vi "CollectorWrap.vi"(7 "Action":T1=enum."Collect") -> ()   [LabVIEW 2013]
uses:
  CollectorWrapAction.ctl
  DoubleSolenoidAction.ctl
  Autonomous/RollerStates.ctl
panel:
  out "error out":errorcluster
  in  "error in":errorcluster
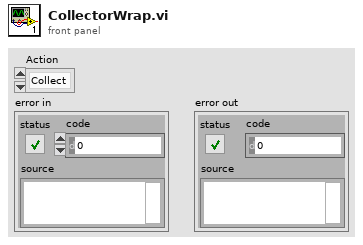
[diagram p1: front panel]
types:
  T1 = typedef "CollectorWrapAction.ctl" = enum16{"PreCollect", "Collect", "Stop"}
  T2 = typedef "DoubleSolenoidAction.ctl" = enum16{"Init", "Middle", "In", "Out"}
  T3 = typedef "RollerStates.ctl" = enum16{"Init", "Off", "Forward", "Reverse"}
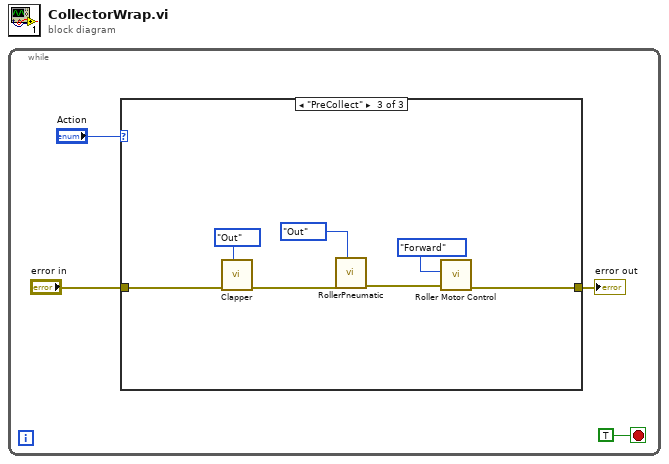
[diagram p0: block diagram]
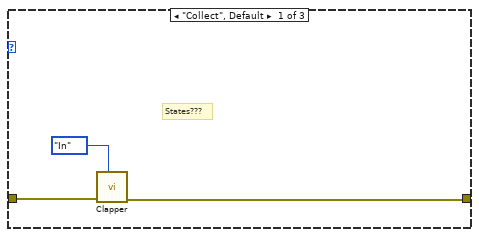
[diagram p2: hidden frame]
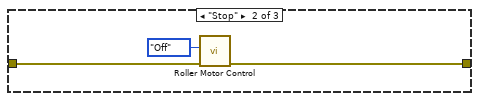
[diagram p3: hidden frame]
diagram:
  n1 = while {
    stop <- TRUE stop-if-true
    n2 = case shown="\"PreCollect\"" "Action" {
      tunnel: "error in" -> [w7 w10 w14]
      tunnel: [w6 w9 w16] -> w1
      frame "Collect", Default {
        # "States???"
        n3 = call "Clapper.vi"("State"=DoubleSolenoidAction."In", "Error in"=w7) -> ("Error out"=w6:errorcluster)  [unwired: 9 in]
      }
      frame "Stop" {
        n4 = call "Roller Motor Control.vi"("Error in"=w10, "RollerState"=RollerStates."Off") -> ("Error out"=w9:errorcluster)  [unwired: 9 in]
      }
      frame "PreCollect" {
        n5 = call "Clapper.vi"("State"=DoubleSolenoidAction."Out", "Error in"=w14) -> ("Error out"=w13:errorcluster)  [unwired: 9 in]
        n6 = call "RollerPneumatic.vi"("State"=DoubleSolenoidAction."Out", "Error in"=w13) -> ("Error out"=w12:errorcluster)  [unwired: 9 in]
        n7 = call "Roller Motor Control.vi"("Error in"=w12, "RollerState"=RollerStates."Forward") -> ("Error out"=w16:errorcluster)  [unwired: 9 in]
      }
    }
    "error out" <- w1
  }
